vi "Tree_insert childs.vi"(6 "Child Position":i32, 7 "Tree.Tag in":string, 8 "error in (no error)":errorcluster, 9 "Child Text":string[](array[string]), 10 "Left Cell String":string, 11 "tree RefNum in":refnum<vi>) -> (0 "error out":errorcluster, 3 "dup tree RefNum":refnum<vi>)   [LabVIEW 2014]
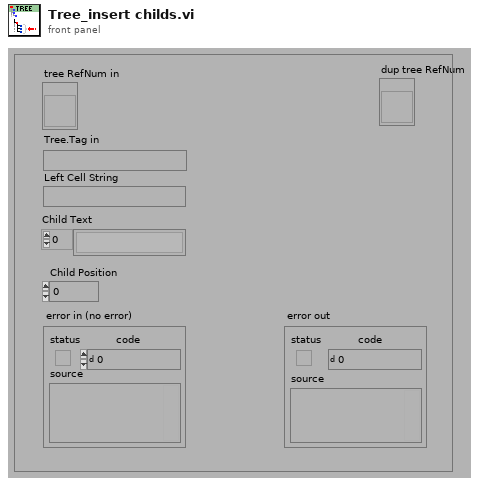
[diagram p1: front panel]
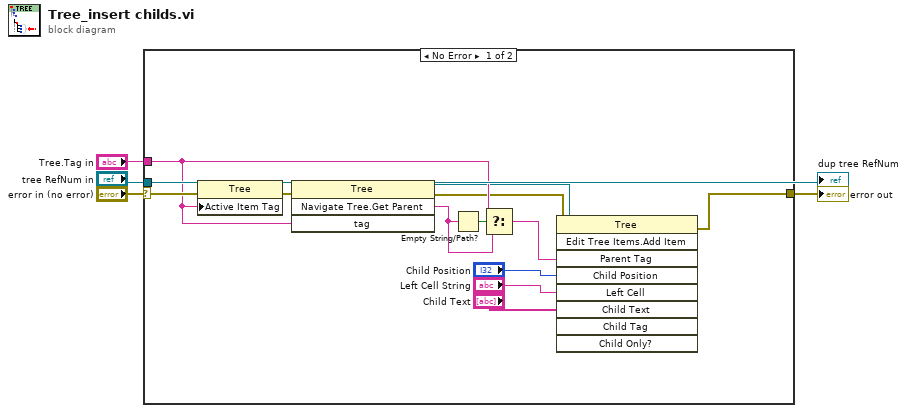
[diagram p0: block diagram]
diagram:
  n1 = case shown="No Error" "error in (no error)" {
    selector: "error in (no error)" -> [w13 w19]
    tunnel: [w16 w19] -> w4
    tunnel: "tree RefNum in" -> [w15 _]
    tunnel: "Tree.Tag in" -> [w11 _]
    frame No Error {
      n2 = property class="Tree"(reference=w15, error in=w13, "Active Item Tag"=w11) -> (reference out=w14:refnum<vi>, error out=w12:errorcluster)
      n3 = invoke class="Tree" method="Navigate Tree.Get Parent"(reference=w14, error in=w12, "tag"=w11) -> (reference out=w8:refnum<vi>, error out=w7:errorcluster, "Navigate Tree:Get Parent"=w17:string)  [unwired: 1 in, 1 out]
      n4 = Empty String/Path?(string/path=w17) -> (empty?=w18:bool)
      n5 = Select(t=w11, s=w18, f=w17) -> (s? t:f=w9:string)
      n6 = invoke class="Tree" method="Edit Tree Items.Add Item"(reference=w8, error in=w7, "Parent Tag"=w9, "Child Position"="Child Position", "Left Cell"="Left Cell String", "Child Text"="Child Text") -> (error out=w16:errorcluster)  [unwired: 3 in, 8 out]
    }
    frame Error {
    }
  }
  "error out" <- w4
  "dup tree RefNum" <- "tree RefNum in"
